vi "Whiskeroscope Main.vi"() -> ()   [LabVIEW 2015]
uses:
  Whiskeroscope Main - States.ctl
  <vilib>/DAQmx/read.llb/DAQmx Read (Analog 2D DBL NChan NSamp).vi
  <vilib>/DAQmx/create/channels.llb/DAQmx Create Channel (AI-Voltage-Basic).vi
  <vilib>/DAQmx/configure/timing.llb/DAQmx Timing (Sample Clock).vi
  <vilib>/Utility/file.llb/Write Delimited Spreadsheet (DBL).vi
  <vilib>/DAQmx/miscellaneous.llb/DAQmx Fill In Error Info.vi
  <vilib>/Analysis/NI_AALBase.lvlib
  <resource>/objmgr/daqmx.rc
panel:
  out "Available":u32
  out "Log Index":i32
  in  "Val 1":dbl=2.55
  in  "Val 2":dbl=2.4
  in  "Save Log Btn":bool
  out "Started":bool
  in  "Stop Btn":bool
  out "Log Data":dbl[][](array[numeric])
  out "Start Time":u32
  out "Data":dbl[][](array[numeric])
  in  "Start Btn":bool
  out "Task":refnum<k21>
  in  "Mean 1":dbl=2.55
  out "Offset 1":dbl format="%.2f"
  in  "Set Ref Btn":bool
  in  "Mean 2":dbl=2.4
  out "Offset 2":dbl format="%.2f"
  out "Force":dbl format="%6.3f"
  out "Distance":dbl format="%6.3f"
  in  "Log File":path=path "C:/Code/Whiskeroscope/Logs/Log.csv"
  in  "Averages":u16=100
  in  "Log Btn":bool=TRUE
  in  "Graph Btn":bool=TRUE
  out "XY Graph":cluster{"X":dbl, "Y":dbl}[](graph)
  out "Amplitude":dbl[][](graph)
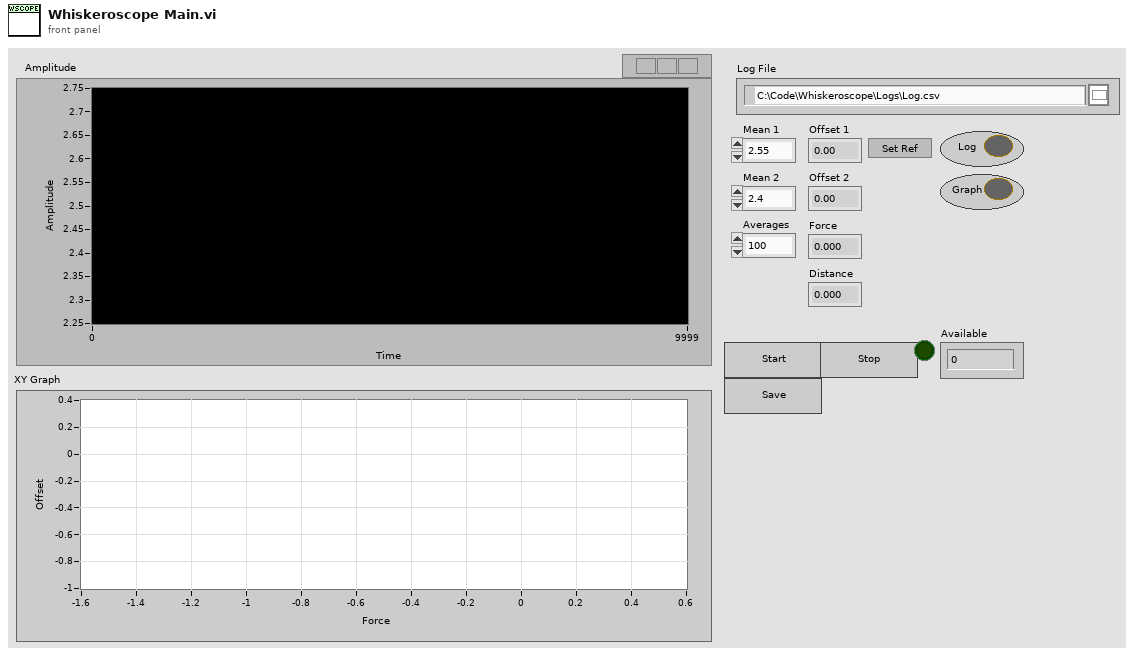
[diagram p1: front panel]
types:
  T1 = typedef "Whiskeroscope Main - States.ctl" = enum16{"Init", "Idle", "Update FP", "Read Data", "Exit"}
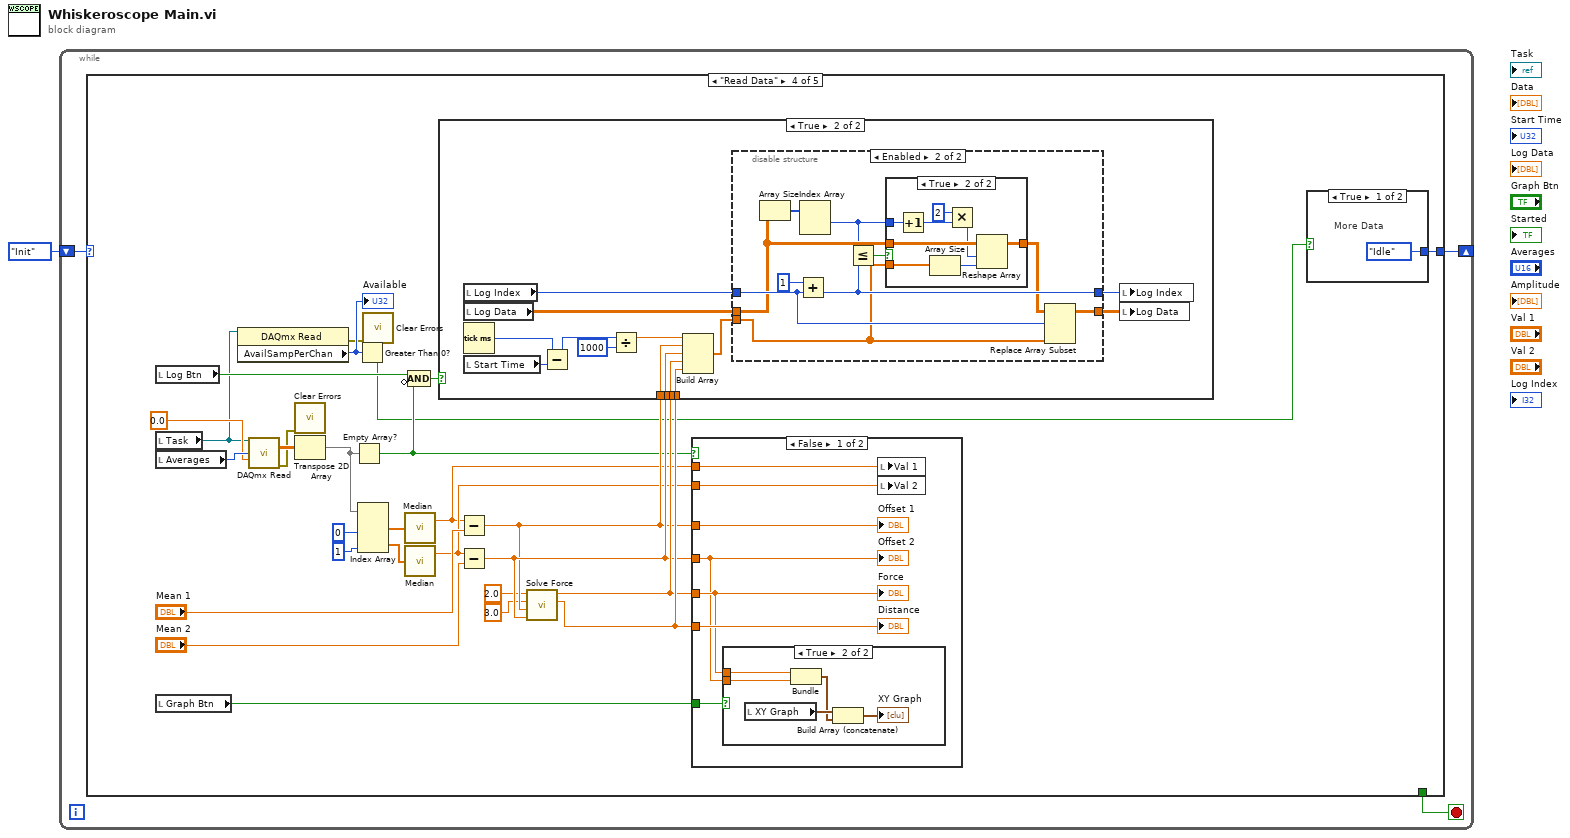
[diagram p0: block diagram]
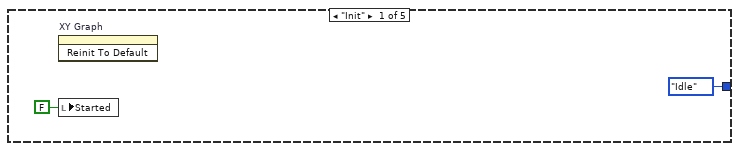
[diagram p2: hidden frame]
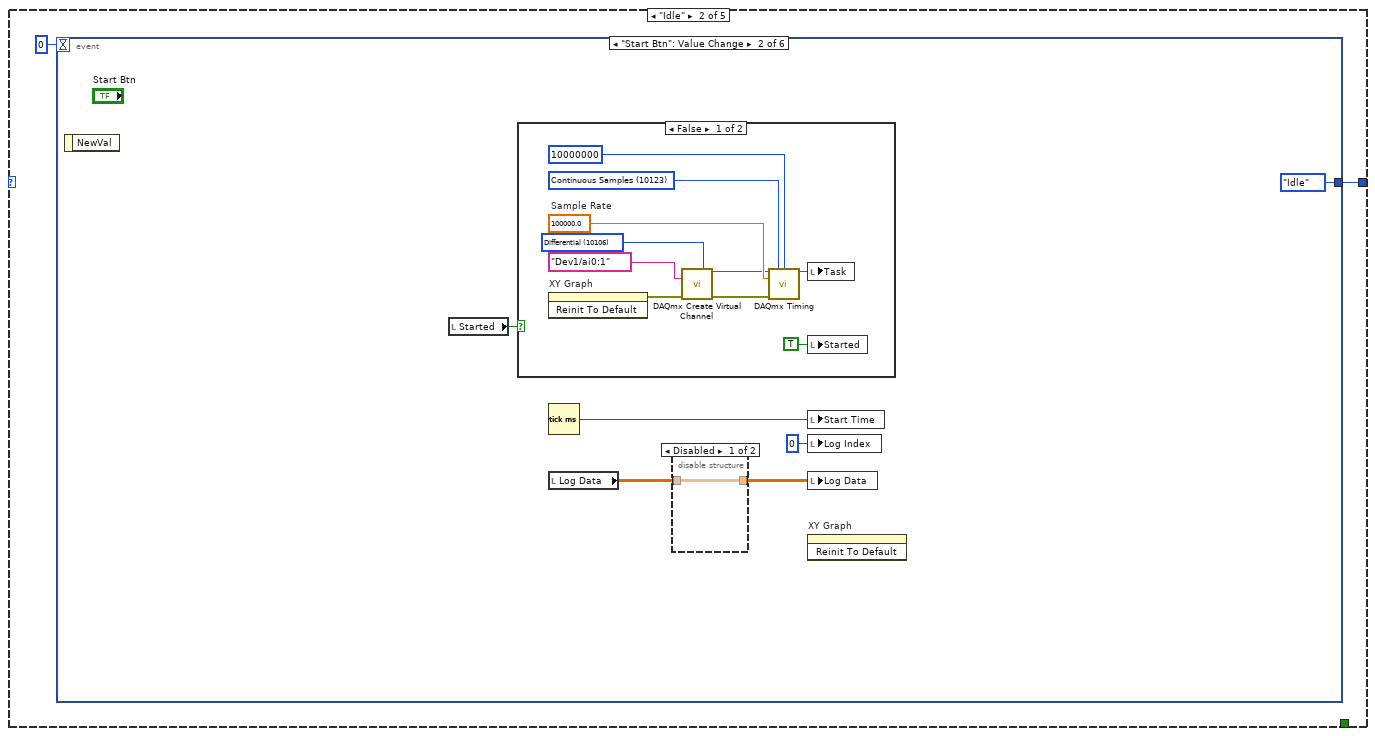
[diagram p3: hidden frame]
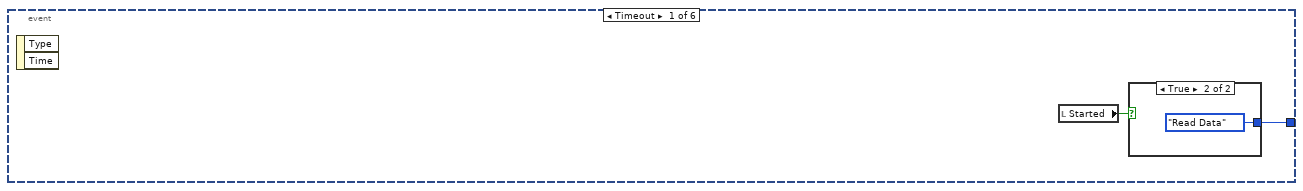
[diagram p4: hidden frame]
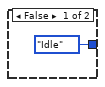
[diagram p5: hidden frame]
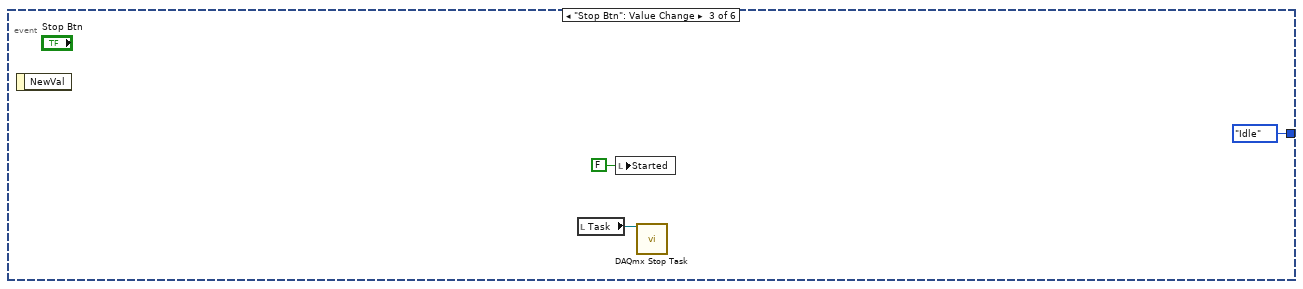
[diagram p8: hidden frame]
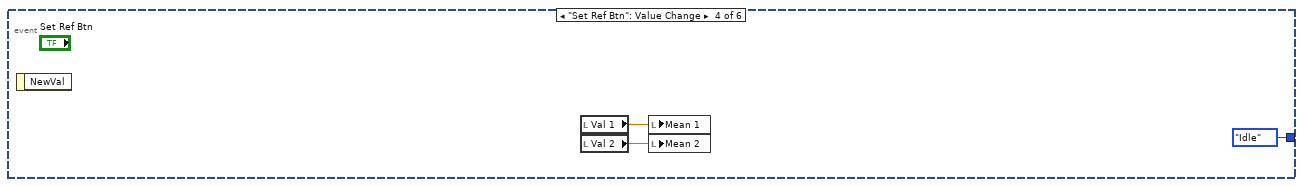
[diagram p9: hidden frame]
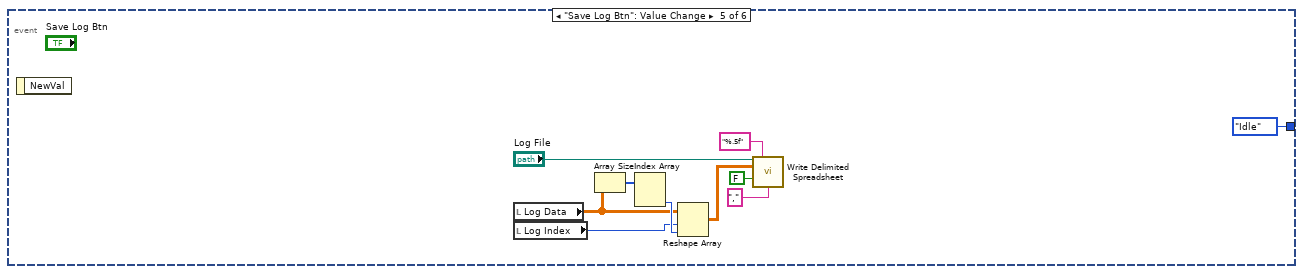
[diagram p10: hidden frame]
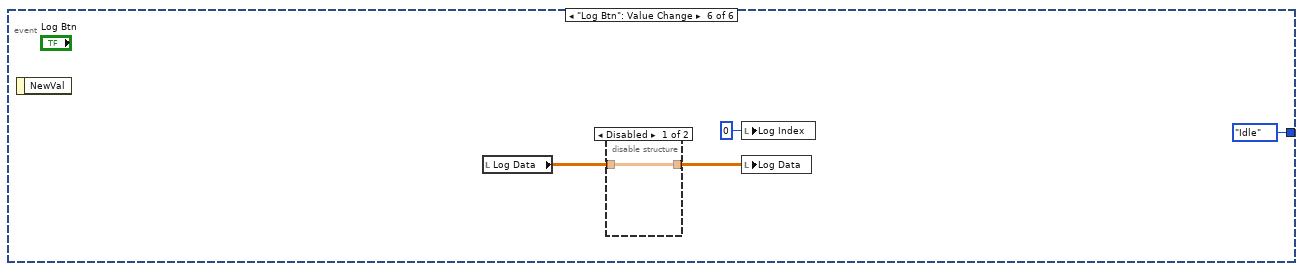
[diagram p11: hidden frame]
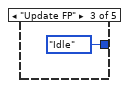
[diagram p13: hidden frame]
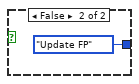
[diagram p14: hidden frame]
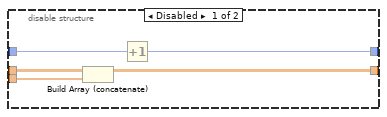
[diagram p18: hidden frame]
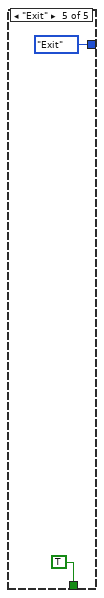
[diagram p20: hidden frame]
diagram:
  n1 = while {
    shift-right: [w3] -> _
    shift-left: Whiskeroscope_Main_-_States."Init" ("States") -> [w4]
    stop <- w2 stop-if-true
    n2 = case shown="\"Read Data\"" w4 {
      tunnel: [Whiskeroscope_Main_-_States."Idle" ("States") w7 Whiskeroscope_Main_-_States."Idle" ("States") w79 Whiskeroscope_Main_-_States."Exit" ("States")] -> w3
      tunnel: [_ _ _ _ TRUE] -> w2
      frame "Init" {
        n3 = invoke on="XY Graph" class="XYGraph (strict)" method="Reinit To Default"() -> ()  [unwired: 3 in, 3 out]
        n4 = local write "Started"(FALSE ("Started")) -> ()
      }
      frame "Idle" {
        n5 = event shown="[1] \"Start Btn\": Value Change" {
          selector: _ -> [_ _ _ _ _ _]
          dyn-events: _ -> [_ _ _ _ _ _]
          timeout: 0 -> [_ _ _ _ _ _]
          tunnel: [w10 Whiskeroscope_Main_-_States."Idle" ("States") Whiskeroscope_Main_-_States."Idle" ("States") Whiskeroscope_Main_-_States."Idle" ("States") Whiskeroscope_Main_-_States."Idle" ("States") Whiskeroscope_Main_-_States."Idle" ("States")] -> w7
          event Timeout {
            n6 = event-data() -> ()  [unwired: 1 in, 2 out]
            n7 = local read "Started"() -> (w9:bool)
            n8 = case shown="True" w9 {
              tunnel: [Whiskeroscope_Main_-_States."Idle" ("States") Whiskeroscope_Main_-_States."Read Data" ("States")] -> w10
              frame False {
              }
              frame True {
              }
            }
          }
          event "Start Btn": Value Change {
            n9 = event-data() -> ()  [unwired: 1 in, 1 out]
            n10 = local read "Started"() -> (w14:bool)
            n11 = case shown="False" w14 {
              frame False {
                w24 = 100000.0  # Sample Rate
                w25 = 10123 items=["Finite Samples"=10178, "Continuous Samples"=10123, "Hardware Timed Single Point"=12522] ("sample mode")
                w21 = 10106 items=["default"=-1, "RSE"=10083, "NRSE"=10078, "Differential"=10106, "Pseudodifferential"=12529] ("input terminal configuration")
                n12 = invoke on="XY Graph" class="XYGraph (strict)" method="Reinit To Default"() -> (error out=w28:errorcluster)  [unwired: 3 in, 2 out]
                n13 = call-poly <vilib>:"DAQmx Create Virtual Channel.vi"("input terminal configuration"=w21, "physical channels"=tag "Dev1/ai0:1", "error in"=w28) -> ("task out"=w22:refnum<k21>, "error out"=w23:errorcluster)  [unwired: 11 in]
                n14 = call-poly <vilib>:"DAQmx Timing.vi"("task/channels in"=w22, "sample mode"=w25, "samples per channel"=10000000, "rate"=w24, "error in"=w23) -> ("task out"=w20:refnum<k21>)  [unwired: 9 in, 1 out]
                n15 = local write "Task"(w20) -> ()
                n16 = local write "Started"(TRUE ("Started")) -> ()
              }
              frame True {
              }
            }
            n17 = Tick Count (ms)() -> (millisecond timer value=w17:u32)
            n18 = local read "Log Data"() -> (w15:dbl[][])
            n19 = disable-structure shown="Disabled" {
              disable-tunnel: [w29 _] -> w16
              disable-tunnel: w15 -> [w29 _]
              frame Disabled {
              }
              frame Enabled {
              }
            }
            n20 = local write "Start Time"(w17) -> ()
            n21 = local write "Log Index"(0 ("Log Index")) -> ()
            n22 = local write "Log Data"(w16) -> ()
            n23 = invoke on="XY Graph" class="XYGraph (strict)" method="Reinit To Default"() -> ()  [unwired: 3 in, 3 out]
          }
          event "Stop Btn": Value Change {
            n24 = event-data() -> ()  [unwired: 1 in, 1 out]
            n25 = local read "Task"() -> (w30:refnum<k21>)
            n26 = local write "Started"(FALSE ("Started")) -> ()
            n27 = call <vilib>:"DAQmx Stop Task.vi"("task/channels in"=w30) -> ()  [unwired: 13 in, 2 out]
          }
          event "Set Ref Btn": Value Change {
            n28 = event-data() -> ()  [unwired: 1 in, 1 out]
            n29 = local read "Val 1"() -> (w34:dbl)
            n30 = local read "Val 2"() -> (w33:dbl)
            n31 = local write "Mean 1"(w34) -> ()
            n32 = local write "Mean 2"(w33) -> ()
          }
          event "Save Log Btn": Value Change {
            n33 = event-data() -> ()  [unwired: 1 in, 1 out]
            n34 = local read "Log Data"() -> (w39:dbl[][])
            n35 = local read "Log Index"() -> (w37:i32)
            n36 = Array Size(array=w39) -> (size(s)=w38:i32[])
            n37 = Index Array(array=w38) -> (element #2=w40:i32)  [unwired: 2 in, 1 out]
            n38 = Reshape Array(w39, w37, w40) -> (w36:dbl[][])
            n39 = call-poly <vilib>:"Write Delimited Spreadsheet.vi"("file path (dialog if empty)"="Log File", "format (%.3f)"="%.5f", "2D data"=w36, "append to file? (F)"=FALSE, "delimiter (\\t)"="," ("delimiter (\\t)")) -> ()  [unwired: 9 in, 2 out]
          }
          event "Log Btn": Value Change {
            n40 = event-data() -> ()  [unwired: 1 in, 1 out]
            n41 = local read "Log Data"() -> (w47:dbl[][])
            n42 = disable-structure shown="Disabled" {
              disable-tunnel: [w50 _] -> w48
              disable-tunnel: w47 -> [w50 _]
              frame Disabled {
              }
              frame Enabled {
              }
            }
            n43 = local write "Log Index"(0 ("Log Index")) -> ()
            n44 = local write "Log Data"(w48) -> ()
          }
        }
      }
      frame "Update FP" {
      }
      frame "Read Data" {
        n45 = local read "Log Btn"() -> (w61:bool)
        n46 = local read "Task"() -> (w56:refnum<k21>)
        n47 = local read "Averages"() -> (w77:u16)
        n48 = local read "Graph Btn"() -> (w65:bool)
        n49 = property class="DAQmx Read"(reference=w56) -> (error out=w53:errorcluster, "AvailSampPerChan"=w55:u32)  [unwired: 1 in, 1 out]
        "Available" <- w55
        n50 = call-poly <vilib>:"DAQmx Read.vi"("task/channels in"=w56, "number of samples per channel"=w77, "timeout"=0.0) -> ("data"=w78:dbl[][], "error out"=w52:errorcluster)  [unwired: 10 in, 1 out]
        n51 = call <vilib>:"Clear Errors.vi"("error in (no error)"=w52) -> ()  [unwired: 5 in, 2 out]
        n52 = Transpose 2D Array(2D array=w78) -> (transposed array=w58:dbl[][])
        n53 = Empty Array?(array=w58) -> (empty?=w57:bool)
        n54 = Greater Than 0?(x=w55) -> (x > 0?=w54:bool)
        n55 = Index Array(array=w58, index (col) #1=0 ("index (row)"), index (col) #2=1 ("index (row)")) -> (element #1=w59:dbl[], element #2=w67:dbl[])  [unwired: 2 in]
        n56 = call <vilib>:"Clear Errors.vi"("error in (no error)"=w53) -> ()  [unwired: 5 in, 2 out]
        n57 = call <vilib>:"Median.vi"("X"=w59) -> ("median"=w63:dbl)  [unwired: 1 out]
        n58 = call <vilib>:"Median.vi"("X"=w67) -> ("median"=w64:dbl)  [unwired: 1 out]
        n59 = Compound Arithmetic op=AND(w61, invert w57) -> (w60:bool)
        n60 = Subtract(x=w63, y="Mean 1") -> (x-y=w73:dbl)
        n61 = Subtract(x=w64, y="Mean 2") -> (x-y=w74:dbl)
        n62 = call "Solve Force.vi"("y2"=w74, "y1"=w73, "x2"=3.0 ("x1"), "x1"=2.0) -> ("D"=w76:dbl, "P"=w75:dbl)  [unwired: 6 in]
        n63 = case shown="True" w60 {
          tunnel: w76 -> [_ w103]
          tunnel: w75 -> [_ w102]
          tunnel: w74 -> [_ w101]
          tunnel: w73 -> [_ w100]
          frame False {
          }
          frame True {
            n64 = local read "Log Index"() -> (w95:i32)
            n65 = local read "Log Data"() -> (w96:dbl[][])
            n66 = Tick Count (ms)() -> (millisecond timer value=w104:u32)
            n67 = local read "Start Time"() -> (w99:u32)
            n68 = Subtract(x=w104, y=w99) -> (x-y=w105:u32)
            n69 = Divide(x=w105, y=u32 1000) -> (x/y=w106:dbl)
            n70 = Build Array(w106, w100, w101, w102, w103) -> (w98:dbl[])
            n71 = disable-structure shown="Enabled" {
              disable-tunnel: w98 -> [w112 w114]
              disable-tunnel: [w111 w122] -> w97
              disable-tunnel: w96 -> [w110 w117]
              disable-tunnel: w95 -> [w109 w120]
              disable-tunnel: [w108 w118] -> w94
              frame Disabled {
                n72 = Build Array (concatenate)(w110, w112) -> (w111:dbl[][])
                n73 = Increment(x=w109) -> (x+1=w108:i32)
              }
              frame Enabled {
                n74 = Array Size(array=w117) -> (size(s)=w121:i32[])
                n75 = Add(x=1, y=w120) -> (x+y=w118:i32)
                n76 = Index Array(array=w121) -> (element #1=w113:i32)  [unwired: 2 in, 1 out]
                n77 = Less Or Equal?(x=w113, y=w118) -> (x <= y?=w115:bool)
                n78 = case shown="True" w115 {
                  tunnel: w117 -> [w123 w131]
                  tunnel: [w123 w130] -> w116
                  tunnel: w114 -> [_ w129]
                  tunnel: w113 -> [_ w126]
                  frame False {
                  }
                  frame True {
                    n79 = Increment(x=w126) -> (x+1=w124:i32)
                    n80 = Array Size(array=w129) -> (size(s)=w128:i32)
                    n81 = Multiply(x=2, y=w124) -> (x*y=w125:i32)
                    n82 = Reshape Array(w131, w125, w128) -> (w130:dbl[][])
                  }
                }
                n83 = Replace Array Subset(array=w116, new element=w114, index (row)=w120) -> (w122:dbl[][])  [unwired: 1 in]
              }
            }
            n84 = local write "Log Index"(w94) -> ()
            n85 = local write "Log Data"(w97) -> ()
          }
        }
        n86 = case shown="False" w57 {
          tunnel: w76 -> [w88 _]
          tunnel: w75 -> [w87 _]
          tunnel: w74 -> [w86 _]
          tunnel: w73 -> [w85 _]
          tunnel: w65 -> [w84 _]
          tunnel: w64 -> [w83 _]
          tunnel: w63 -> [w82 _]
          frame False {
            n87 = case shown="True" w84 {
              tunnel: w86 -> [_ w90]
              tunnel: w87 -> [_ w89]
              frame False {
              }
              frame True {
                n88 = local read "XY Graph"() -> (w93:cluster{"X":dbl, "Y":dbl}[])
                n89 = Bundle("P"=w89, w90) -> (w91:cluster{"P":dbl, dbl})  [unwired: 1 in]
                n90 = Build Array (concatenate)(w93, w91) -> (→"XY Graph":cluster{"P":dbl, "Y":dbl}[])
              }
            }
            n91 = local write "Val 1"(w82) -> ()
            n92 = local write "Val 2"(w83) -> ()
            "Offset 1" <- w85
            "Offset 2" <- w86
            "Force" <- w87
            "Distance" <- w88
          }
          frame True {
          }
        }
        n93 = case shown="True" w54 {
          tunnel: [Whiskeroscope_Main_-_States."Idle" ("States") Whiskeroscope_Main_-_States."Update FP" ("States")] -> w79
          frame True {
            # "More Data"
          }
          frame False {
          }
        }
      }
      frame "Exit" {
      }
    }
  }
